vi "Autoscan_CheckEmitter.vi"(0 "String in":refnum<vi>, 1 "reference 5":refnum<vi>, 2 "IntGraph Refnum":refnum<vi>, 3 "reference 6":refnum<vi>, 4 "reference 7":refnum<vi>, 5 "reference 8":refnum<vi>, 6 "reference 9":refnum<vi>, 7 "error in (no error)":errorcluster, 8 "reference 4":refnum<vi>, 9 "reference 10":refnum<vi>, 10 "reference 3":refnum<vi>, 11 "reference 11":refnum<vi>, 12 "reference in":refnum<vi>, 13 "lowerbright":dbl=40000.0, 14 "upperbright":dbl=8000000.0, 16 "Numeric in":i32, 18 "Cluster":T1) -> (19 "Autoscan Emitter Position":dbl[](array[numeric]), 20 "Numeric out":i32, 21 "Array":dbl[][](array[numeric]), 22 "Emitter # out":i32, 23 "Boolean":bool, 24 "Ystored":dbl=45.85, 25 "Zstored":dbl=48.40147356000009 format="%.3g", 26 "Xstored":dbl=51.85, 27 "error out":errorcluster)   [LabVIEW 2023]
uses:
  <vilib>/Analysis/baseanly.llb/Mean (DBL).vi
  <vilib>/Analysis/NI_AALBase.lvlib
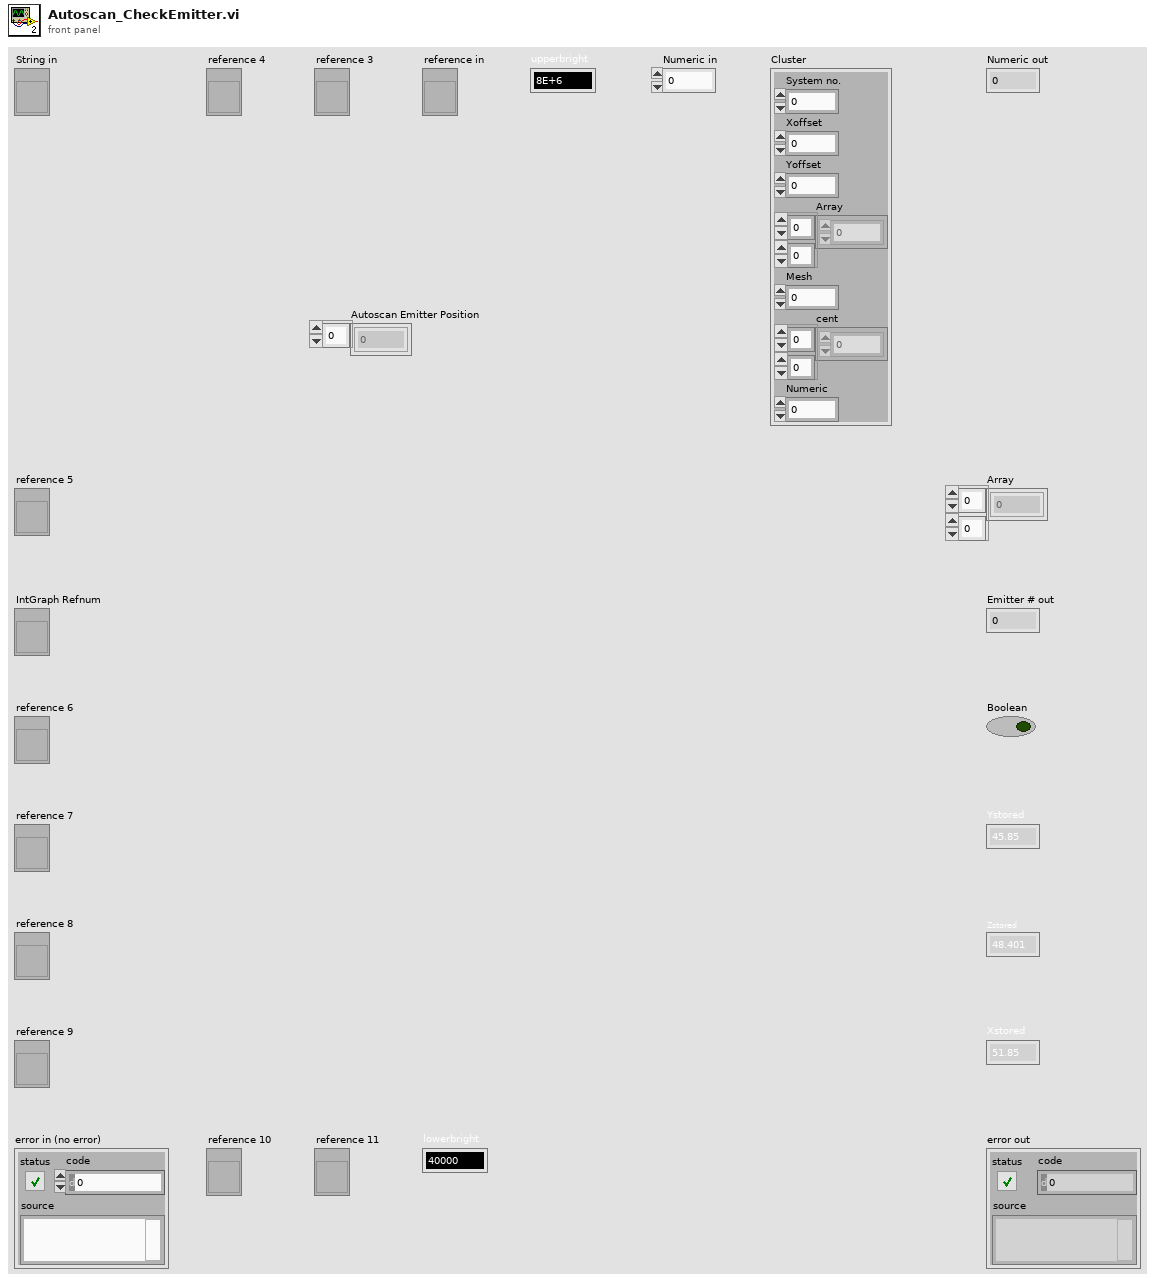
[diagram p1: front panel]
types:
  T1 = cluster{"System no.":i32, "Xoffset":dbl, "Yoffset":dbl, "Array":dbl[][], "Mesh":dbl, "cent":i32[][], "Numeric":i32}
  T2 = enum16{"Maximum", "End Position", "Center of scan"}
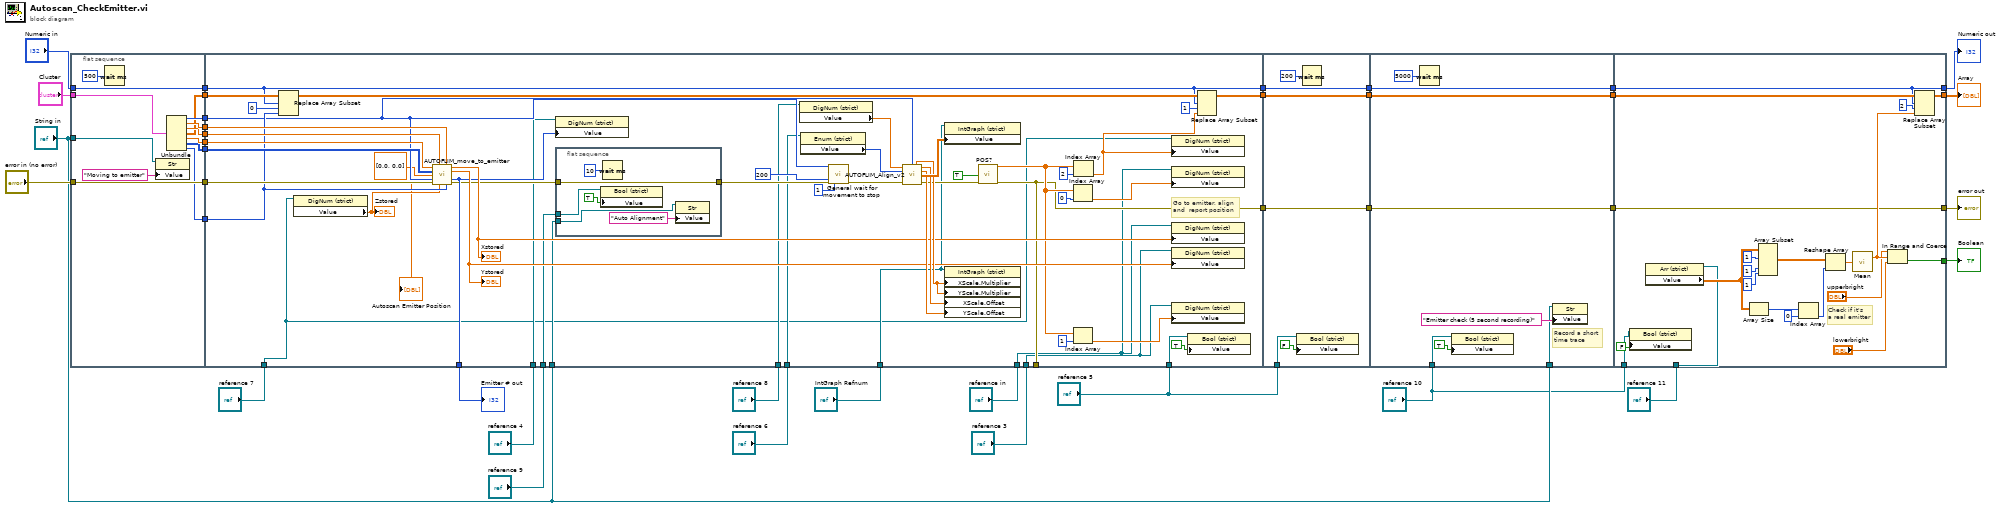
[diagram p0: block diagram]
diagram:
  n1 = flat-sequence {
    tunnel: "Numeric in" -> [w51]
    tunnel: [w50] -> w38
    tunnel: [w41] -> w37
    tunnel: [w46] -> w36
    tunnel: [w40] -> w35
    tunnel: [w42] -> w34
    tunnel: [w45] -> w33
    tunnel: [w44] -> w32
    tunnel: [w43] -> w31
    tunnel: [w51] -> w30
    tunnel: "error in (no error)" -> [w50]
    tunnel: "Cluster" -> [w47]
    tunnel: "String in" -> [w39]
    tunnel: [w63] -> _
    tunnel: [w72] -> w29
    tunnel: [w71] -> w28
    tunnel: [w69] -> w13
    tunnel: w38 -> [w102]
    tunnel: w37 -> [w101]
    tunnel: w36 -> [w70]
    tunnel: w35 -> [w76]
    tunnel: w34 -> [w100]
    tunnel: w33 -> [w99]
    tunnel: w32 -> [w98]
    tunnel: w31 -> [w78]
    tunnel: w30 -> [w71]
    tunnel: [w63] -> w27
    tunnel: "reference 4" -> [w62]
    tunnel: "reference 5" -> [w61]
    tunnel: "reference 6" -> [w60]
    tunnel: "IntGraph Refnum" -> [w59]
    tunnel: "reference in" -> [w58]
    tunnel: "reference 3" -> [w57]
    tunnel: "reference 8" -> [w56]
    tunnel: "reference 9" -> [w55]
    tunnel: "String in" -> [w54]
    tunnel: "reference 7" -> [w53]
    tunnel: [w112] -> w26
    tunnel: w29 -> [w112]
    tunnel: [w111] -> w25
    tunnel: w28 -> [w111]
    tunnel: [w110] -> w24
    tunnel: w27 -> [w110]
    tunnel: "reference 5" -> [w109]
    tunnel: [w120] -> w23
    tunnel: w26 -> [w120]
    tunnel: [w119] -> w22
    tunnel: w25 -> [w119]
    tunnel: [w117] -> w21
    tunnel: w24 -> [w117]
    tunnel: "reference 10" -> [w116]
    tunnel: "String in" -> [w115]
    tunnel: [w131] -> w14
    tunnel: w23 -> [w133]
    tunnel: w22 -> [w127]
    tunnel: [w132] -> w15
    tunnel: [w127] -> w18
    tunnel: [w126] -> w17
    tunnel: w21 -> [w126]
    tunnel: "reference 11" -> [w125]
    tunnel: "reference 10" -> [w124]
    frame #0 {
      n2 = Wait (ms)(milliseconds to wait=u32 500) -> ()  [unwired: 1 out]
      n3 = property class="Str"(reference=w39, "Value"="Moving to emitter") -> ()  [unwired: 1 in, 2 out]
      n4 = Unbundle(w47) -> ("System no."=w46:i32, "Xoffset"=w45:dbl, "Yoffset"=w44:dbl, "Array"=w43:dbl[][], "Mesh"=w42:dbl, "cent"=w41:i32[][], "Numeric"=w40:i32)
    }
    frame #1 {
      # "Go to emitter, align \nand  report position"
      n5 = Replace Array Subset(array=w78, new element=w76, index (row)=w71, index (col)=0 ("disabled index (col)")) -> (w73:dbl[][])
      n6 = property class="DigNum (strict)"(reference=w53) -> ("Value"=w64:dbl)  [unwired: 1 in, 2 out]
      "Zstored" <- w64
      n7 = call "AUTOFLIM_move_to_emitter.vi"("Mesh"=w100, "YScale.Offset"=w98, "XScale.Offset"=w99, "cent"=w101, "Drift"=dbl[] [0.0, 0.0] ("drift vector"), "System no."=w70, "error in (no error)"=w102, "Z"=w64, "Emitter # in"=w76) -> ("Numeric 2"=w90:dbl, "Numeric"=w91:dbl, "Emitter # out"=w69:i32, "Autoscan Emitter Position"=→"Autoscan Emitter Position":dbl[], "error out"=w66:errorcluster)  [unwired: 2 in]
      "Xstored" <- w90
      "Ystored" <- w91
      n8 = property class="DigNum (strict)"(reference=w62, "Value"=w69) -> ()  [unwired: 1 in, 2 out]
      n9 = flat-sequence {
        tunnel: w66 -> [w107]
        tunnel: [w107] -> w65
        tunnel: w55 -> [w104]
        tunnel: w54 -> [w103]
        frame #0 {
          n10 = property class="Bool (strict)"(reference=w104, "Value"=TRUE ("Motion")) -> ()  [unwired: 1 in, 2 out]
          n11 = Wait (ms)(milliseconds to wait=u32 10) -> ()  [unwired: 1 out]
          n12 = property class="Str"(reference=w103, "Value"="Auto Alignment") -> ()  [unwired: 1 in, 2 out]
        }
      }
      n13 = property class="DigNum (strict)"(reference=w56) -> ("Value"=w67:dbl)  [unwired: 1 in, 2 out]
      n14 = property class="Enum (strict)"(reference=w60) -> ("Value"=w95:T2)  [unwired: 1 in, 2 out]
      n15 = call "General wait for movement to stop.vi"("System no."=w70, "Additional wait time, ms"=u32 200, "error in"=w65, "Polling cycle \ntime, ms"=u32 1 ("Polling cycle \ntime, ms")) -> ("error out"=w89:errorcluster)  [unwired: 4 in, 11 out]
      n16 = call "AUTOFLIM_Align_v2.vi"("Z Scan Range"=w67, "System no."=w70, "Scan Termination"=w95, "error in (no error)"=w89) -> ("Mesh out"=w92:dbl, "Numeric 2"=w94:dbl, "Numeric"=w93:dbl, "Alignment Graph"=w96:dbl[][], "error out"=w82:errorcluster)  [unwired: 6 in, 1 out]
      n17 = property class="IntGraph (strict)"(reference=w59, "Value"=w96) -> ()  [unwired: 1 in, 2 out]
      n18 = property on="Property Node" class="IntGraph (strict)"(reference=w59, "XScale.Multiplier"=w92, "YScale.Multiplier"=w92, "XScale.Offset"=w94, "YScale.Offset"=w93) -> ()  [unwired: 1 in, 2 out]
      n19 = call "POS?.vi"("All axes?"=TRUE, "error in"=w82) -> ("Position"=w84:dbl[], "error out"=w63:errorcluster)  [unwired: 3 in, 13 out]
      n20 = Index Array(array=w84, index=0) -> (element=w81:dbl)
      n21 = Index Array(array=w84, index=1) -> (element=w80:dbl)
      n22 = Index Array(array=w84, index=2) -> (element=w74:dbl)
      n23 = property class="DigNum (strict)"(reference=w53, "Value"=w74) -> ()  [unwired: 1 in, 2 out]
      n24 = property class="DigNum (strict)"(reference=w58, "Value"=w81) -> ()  [unwired: 1 in, 2 out]
      n25 = property class="DigNum (strict)"(reference=w58, "Value"=w90) -> ()  [unwired: 1 in, 2 out]
      n26 = property class="DigNum (strict)"(reference=w57, "Value"=w91) -> ()  [unwired: 1 in, 2 out]
      n27 = property class="DigNum (strict)"(reference=w57, "Value"=w80) -> ()  [unwired: 1 in, 2 out]
      n28 = property class="Bool (strict)"(reference=w61, "Value"=TRUE ("Empty memory")) -> ()  [unwired: 1 in, 2 out]
      n29 = Replace Array Subset(array=w73, new element=w74, index (row)=w71, index (col)=1 ("disabled index (col)")) -> (w72:dbl[][])
    }
    frame #2 {
      n30 = property class="Bool (strict)"(reference=w109, "Value"=FALSE ("Empty memory")) -> ()  [unwired: 1 in, 2 out]
      n31 = Wait (ms)(milliseconds to wait=u32 200) -> ()  [unwired: 1 out]
    }
    frame #3 {
      # "Record a short\ntime trace"
      n32 = Wait (ms)(milliseconds to wait=u32 5000) -> ()  [unwired: 1 out]
      n33 = property class="Bool (strict)"(reference=w116, "Value"=TRUE ("Record stab")) -> ()  [unwired: 1 in, 2 out]
      n34 = property class="Str"(reference=w115, "Value"="Emitter check (5 second recording)") -> ()  [unwired: 1 in, 2 out]
    }
    frame #4 {
      # "Check if it's \na real emitter"
      n35 = property class="Bool (strict)"(reference=w124, "Value"=FALSE) -> ()  [unwired: 1 in, 2 out]
      n36 = property class="Arr (strict)"(reference=w125) -> ("Value"=w139:dbl[][])  [unwired: 1 in, 2 out]
      n37 = Array Size(array=w139) -> (size(s)=w138:i32[])
      n38 = Array Subset(array=w139, index (row)=1 ("index"), index (col)=1 ("index"), length (col)=1 ("length")) -> (w140:dbl[][])  [unwired: 1 in]
      n39 = Index Array(array=w138, index=0) -> (element=w136:i32)
      n40 = Reshape Array(w140, w136) -> (w135:dbl[])
      n41 = call-poly <vilib>:"Mean.vi"("X"=w135) -> ("mean"=w130:dbl)  [unwired: 1 out]
      n42 = In Range and Coerce(upper limit="upperbright", x=w130, lower limit="lowerbright") -> (In Range?=w131:bool)  [unwired: 1 out]
      n43 = Replace Array Subset(array=w133, new element=w130, index (row)=w127, index (col)=2 ("disabled index (col)")) -> (w132:dbl[][])
    }
  }
  "Numeric out" <- w18
  "error out" <- w17
  "Array" <- w15
  "Boolean" <- w14
  "Emitter # out" <- w13
